vi "Actuators_n_Sensor_Global.vi"() -> ()   [LabVIEW 2019]
panel:
  in  "Reset Encoder":bool
  out "Right Encoder":dbl
  out "Left Encoder":dbl
  out "TurretDegrees":dbl
  out "LL Mode":dbl
  out "LL LED Status":dbl
  out "LL Y":dbl
  out "LL X":dbl
  out "LL in Range":bool
  out "LL True Target":bool
  out "PTOSolenoid":bool
  out "ClimberSolenoid":bool
  out "IntakeSolenoid":bool
  out "HoodOutput":dbl
  out "JoystickRumble":dbl
  out "TurretEncoder":dbl
  out "TurretOutput":dbl
  out "IndexerOutput":dbl
  out "SpindexerOutput":dbl
  out "IntakeOutput":dbl
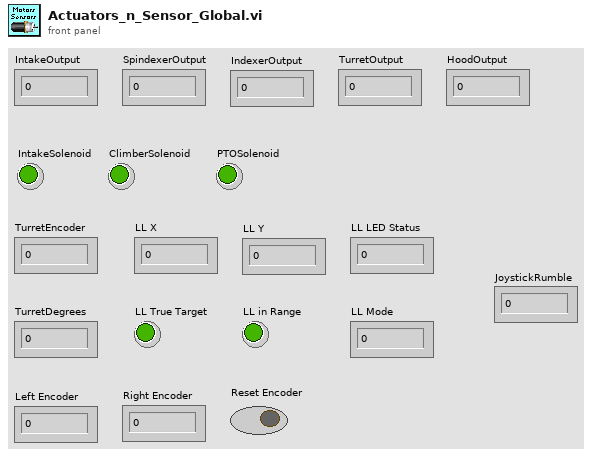
[diagram p1: front panel]
diagram:
